vi "ApplicationConfigReadIniFile.vi"(8 "error in (no error)":errorcluster, 11 "IniFilePath":path) -> (0 "error out":errorcluster, 3 "ApplicationConfig":T1)   [LabVIEW 2013]
uses:
  Ctrls/ApplicationConfig.ctl
  Ctrls/MessageHandlerConfig.ctl
  EnumApplicationConfigIniSections.ctl
  EnumApplicationConfigIniKeys.ctl
  <vilib>/Utility/config.llb/NI_LVConfig.lvlib
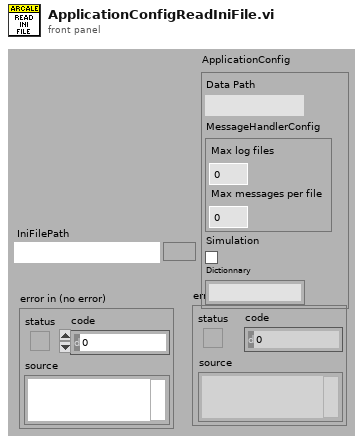
[diagram p1: front panel]
types:
  T1 = typedef "ApplicationConfig.ctl" = cluster{"Data Path":path, "MessageHandlerConfig":T2, "Simulation":bool, "Dictionnary":string}
  T2 = typedef "MessageHandlerConfig.ctl" = cluster{"Max log files":u32, "Max messages per file":u32}
  T3 = typedef "EnumApplicationConfigIniKeys.ctl" = enum16{"Simulation", "Data path", "Max LOG files", "Max message per LOG file", "Dictionnary"}
  T4 = typedef "EnumApplicationConfigIniSections.ctl" = enum16{"GLOBAL", "LOG", "LOCALIZATION"}
  T5 = typedef "NI_LVConfig.lvlib/Config Data RefNum.ctl" = refnum<k1>
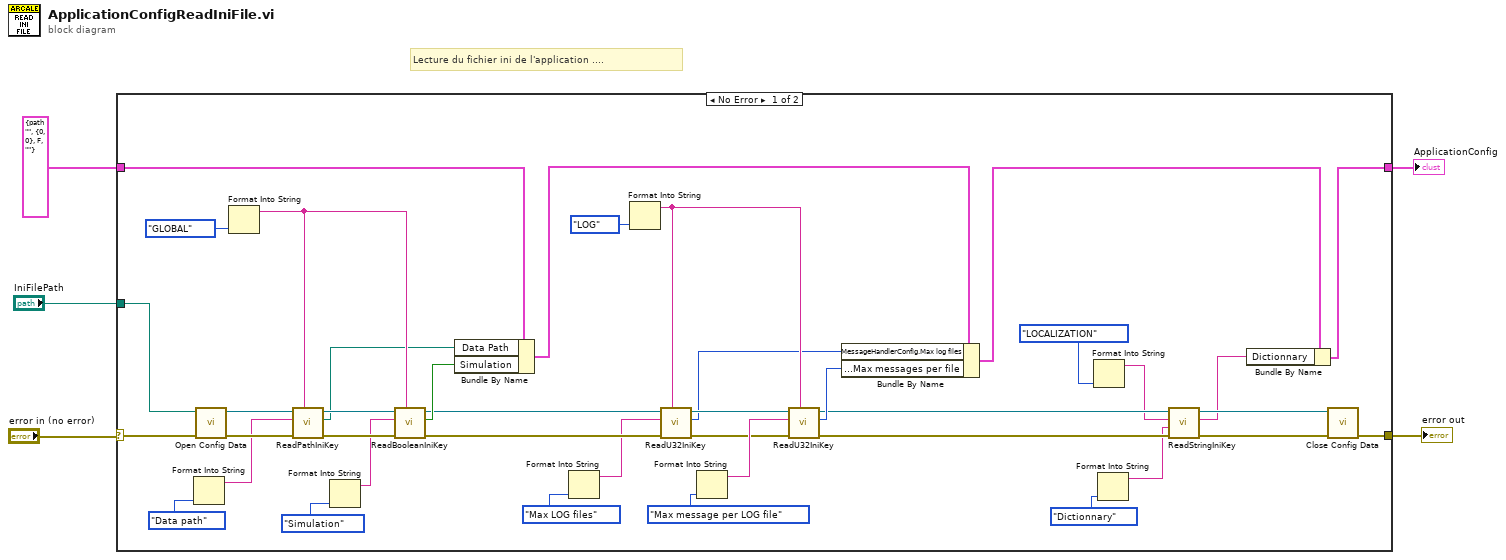
[diagram p0: block diagram]
diagram:
  # "Lecture du fichier ini de l'application ...."
  n1 = case shown="No Error" "error in (no error)" {
    selector: "error in (no error)" -> [w45 w46]
    tunnel: "IniFilePath" -> [w44 _]
    tunnel: T1 {"Data Path"=path "", "MessageHandlerConfig"={"Max log files"=0, "Max messages per file"=0}, "Simulation"=FALSE, "Dictionnary"=""} ("ApplicationConfig") -> [w31 w47]
    tunnel: [w7 w47] -> w2
    tunnel: [w17 w46] -> w1
    frame No Error {
      n2 = Format Into String(EnumApplicationConfigIniKeys."Data path" ("Clé")) -> (resulting string=w39:string)  [unwired: 3 in, 1 out]
      n3 = call <vilib>:"Open Config Data.vi"("error in (no error)"=w45, "configuration file path"=w44) -> ("error out"=w43:errorcluster, "refnum"=w42:T5)  [unwired: 7 in, 1 out]
      n4 = Format Into String(EnumApplicationConfigIniSections."GLOBAL" ("Section")) -> (resulting string=w36:string)  [unwired: 3 in, 1 out]
      n5 = call "ReadPathIniKey.vi"("Section"=w36, "error in (no error)"=w43, "Key"=w39, "refnum In"=w42) -> ("error out"=w38:errorcluster, "Value"=w33:path, "refnum out"=w37:T5)  [unwired: 5 in]
      n6 = Format Into String(EnumApplicationConfigIniKeys."Simulation" ("Clé")) -> (resulting string=w34:string)  [unwired: 3 in, 1 out]
      n7 = call "ReadBooleanIniKey.vi"("Section"=w36, "error in (no error)"=w38, "Key"=w34, "refnum In"=w37) -> ("error out"=w30:errorcluster, "Value"=w32:bool, "refnum out"=w29:T5)  [unwired: 5 in]
      n8 = Bundle By Name(cluster=w31, "Data Path"=w33, "Simulation"=w32) -> (w25:T1)
      n9 = Format Into String(EnumApplicationConfigIniKeys."Max LOG files" ("Clé")) -> (resulting string=w26:string)  [unwired: 3 in, 1 out]
      n10 = Format Into String(EnumApplicationConfigIniSections."LOG" ("Section")) -> (resulting string=w20:string)  [unwired: 3 in, 1 out]
      n11 = call "ReadU32IniKey.vi"("Section"=w20, "error in (no error)"=w30, "Key"=w26, "refnum In"=w29) -> ("error out"=w22:errorcluster, "Value"=w19:u32, "refnum out"=w21:T5)  [unwired: 5 in]
      n12 = Format Into String(EnumApplicationConfigIniKeys."Max message per LOG file" ("Clé")) -> (resulting string=w23:string)  [unwired: 3 in, 1 out]
      n13 = call "ReadU32IniKey.vi"("Section"=w20, "error in (no error)"=w22, "Key"=w23, "refnum In"=w21) -> ("error out"=w15:errorcluster, "Value"=w18:u32, "refnum out"=w13:T5)  [unwired: 5 in]
      n14 = Bundle By Name(cluster=w25, "MessageHandlerConfig.Max log files"=w19, "MessageHandlerConfig.Max messages per file"=w18) -> (w24:T1)
      n15 = Format Into String(EnumApplicationConfigIniSections."LOCALIZATION" ("Section")) -> (resulting string=w10:string)  [unwired: 3 in, 1 out]
      n16 = Format Into String(EnumApplicationConfigIniKeys."Dictionnary" ("Clé")) -> (resulting string=w8:string)  [unwired: 3 in, 1 out]
      n17 = call "ReadStringIniKey.vi"("error in (no error)"=w15, "Key"=w8, "Section"=w10, "refnum In"=w13) -> ("error out"=w14:errorcluster, "Value"=w6:string, "refnum out"=w12:T5)  [unwired: 5 in]
      n18 = Bundle By Name(cluster=w24, "Dictionnary"=w6) -> (w7:T1)
      n19 = call <vilib>:"Close Config Data.vi"("error in (no error)"=w14, "refnum"=w12) -> ("error out"=w17:errorcluster)  [unwired: 8 in, 1 out]
    }
    frame Error {
    }
  }
  "error out" <- w1
  "ApplicationConfig" <- w2
